vi "Live Image Test.vi"() -> ()   [LabVIEW 2017]
uses:
  <vilib>/vision/NI_Vision_Development_Module.lvlib
panel:
  in  "IP Address":string="192.168.0.90"
  out "HSL Image":T1(plugin-control)
  in  "Debug":bool
  out "Mono Image":T1(plugin-control)
  in  "Track":bool
  in  "Tracking":enum16{"None", "Color", "Circle", "Rect"}(ring)
  in  "Camera Op":T2(ring)=enum."JPG-CGI"
  in  "Acquire Params":T3={"fps"=10, "Compress"=30, "X Size"=320, "Y Size"=240, "Color?"=TRUE, "Rotation"=enum."0"}
  out "Waveform Chart":u32(graph)
  out "dT":u32
  in  "stop":bool
  out "Image":T1(plugin-control)
  out "Objects":i32
  # "Camera"
  # "Vision"
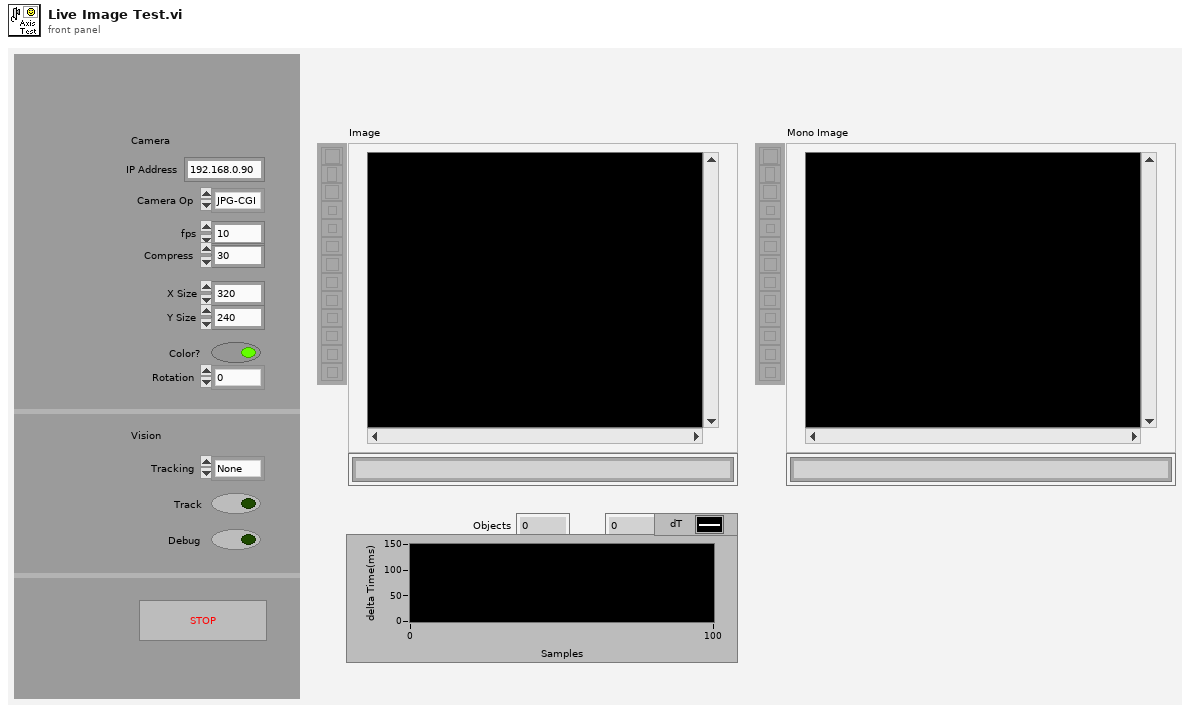
[diagram p1: front panel]
types:
  T1 = typedef "IMAQ Image.ctl" = refnum<image>
  T2 = enum16{"MJPG", "JPG", "JPG-CGI", "BMP", "BMP-CGI"}
  T3 = cluster{"fps":i32, "Compress":i32, "X Size":i32, "Y Size":i32, "Color?":bool, "Rotation":enum16{"0", "90", "180", "270"}}
  T4 = typedef "Image Type" = u32
  T5 = typedef "IMAQ ExtractCurvesCurve.ctl" = cluster{"Points":cluster{"X":dbl, "Y":dbl}[], "Closed?":bool, "Curve Length":dbl, "Min Edge Strength":dbl, "Max Edge Strength":dbl, "Average Edge Strength":dbl}
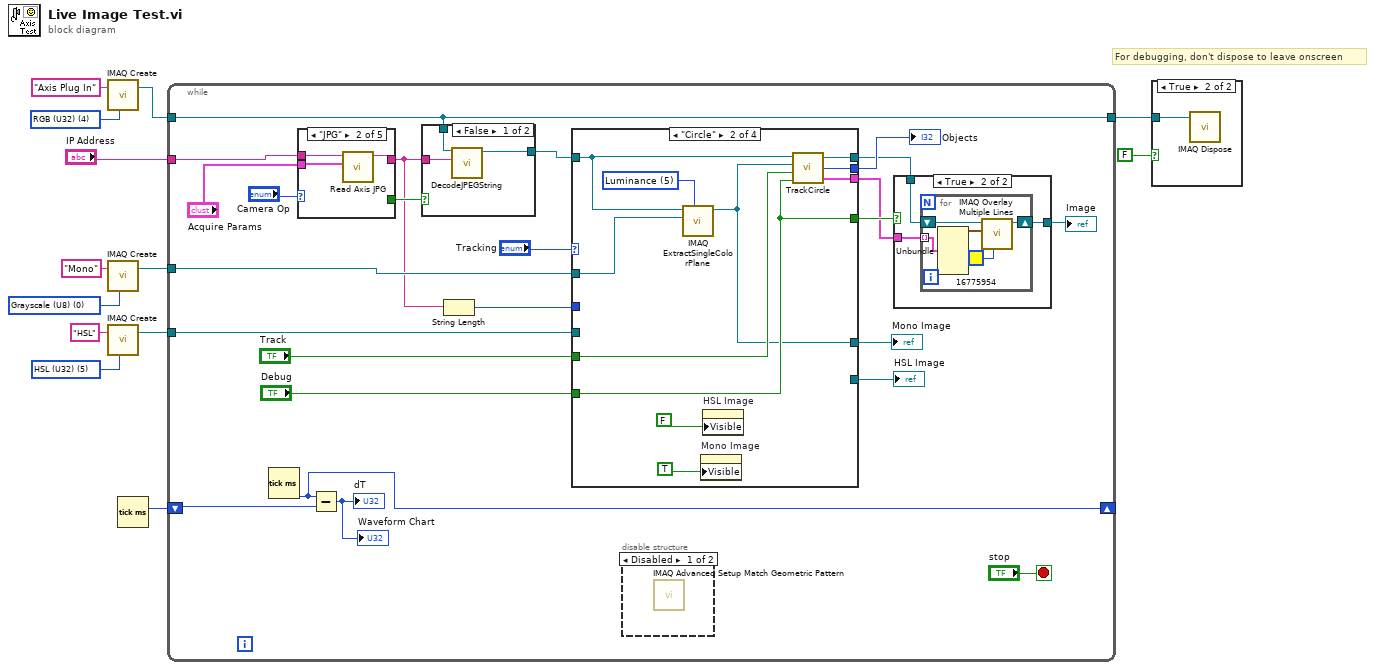
[diagram p0: block diagram]
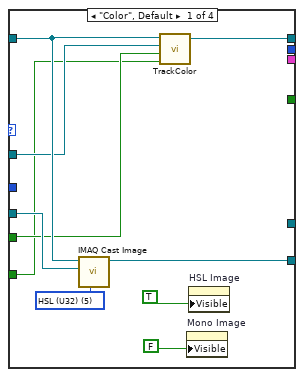
[diagram p5: hidden frame]
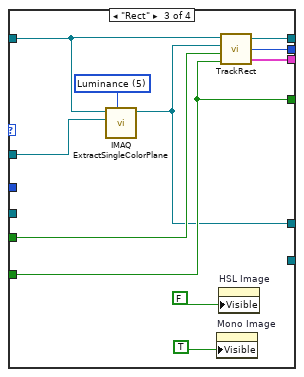
[diagram p6: hidden frame]
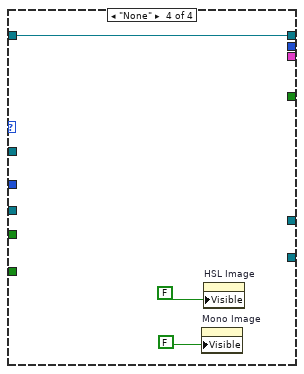
[diagram p7: hidden frame]
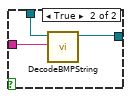
[diagram p8: hidden frame]
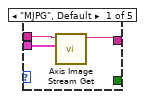
[diagram p9: hidden frame]
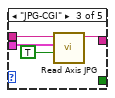
[diagram p10: hidden frame]
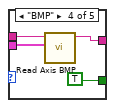
[diagram p11: hidden frame]
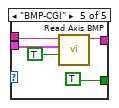
[diagram p12: hidden frame]
diagram:
  w2 = T4 5 items=["Grayscale (U8)", "Grayscale (I16)", "Grayscale (SGL)", "Complex (CSG)", "RGB (U32)", "HSL (U32)", "RGB (U64)"] ("Image Type")
  w6 = T4 0 items=["Grayscale (U8)", "Grayscale (I16)", "Grayscale (SGL)", "Complex (CSG)", "RGB (U32)", "HSL (U32)", "RGB (U64)"] ("Image Type")
  w7 = T4 4 items=["Grayscale (U8)", "Grayscale (I16)", "Grayscale (SGL)", "Complex (CSG)", "RGB (U32)", "HSL (U32)", "RGB (U64)"] ("Image Type")
  # "For debugging, don't dispose to leave onscreen"
  n1 = call "IMAQ Create"("Image Name"="Axis Plug In", "Image Type"=w7) -> ("New Image"=w12:T1)  [unwired: 3 in, 1 out]
  n2 = call "IMAQ Create"("Image Name"="Mono", "Image Type"=w6) -> ("New Image"=w4:T1)  [unwired: 3 in, 1 out]
  n3 = call "IMAQ Create"("Image Name"="HSL", "Image Type"=w2) -> ("New Image"=w1:T1)  [unwired: 3 in, 1 out]
  n4 = Tick Count (ms)() -> (millisecond timer value=w11:u32)
  n5 = while {
    tunnel: w12 -> [w33]
    shift-right: [w35] -> _
    shift-left: w11 -> [w36]
    tunnel: [w33] -> w10
    tunnel: "IP Address" -> [w30]
    tunnel: w4 -> [w27]
    tunnel: w1 -> [w14]
    stop <- "stop" stop-if-true
    n6 = Tick Count (ms)() -> (millisecond timer value=w35:u32)
    n7 = case shown="\"JPG\"" "Camera Op" {
      tunnel: w30 -> [w90 w93 w97 w101 w105]
      tunnel: [w89 w92 w96 w100 w106] -> w23
      tunnel: "Acquire Params" -> [w88 w91 w95 w99 w104]
      tunnel: [_ _ _ TRUE TRUE] -> w31
      frame "MJPG", Default {
        n8 = call <vilib>:"Axis Image Stream Get.vi"("Acquire Params"=w88, "IP Address"=w90) -> ("Raw Image Data"=w89:string)  [unwired: 9 in]
      }
      frame "JPG" {
        n9 = call <vilib>:"Read Axis JPG.vi"("Acquire Params"=w91, "address"=w93) -> ("Raw Image Data"=w92:string)  [unwired: 8 in, 1 out]
      }
      frame "JPG-CGI" {
        n10 = call <vilib>:"Read Axis JPG.vi"("CGI?"=TRUE, "Acquire Params"=w95, "address"=w97) -> ("Raw Image Data"=w96:string)  [unwired: 7 in, 1 out]
      }
      frame "BMP" {
        n11 = call <vilib>:"Read Axis BMP.vi"("Acquire Params"=w99, "address"=w101) -> ("Raw Image Data"=w100:string)  [unwired: 8 in, 1 out]
      }
      frame "BMP-CGI" {
        n12 = call <vilib>:"Read Axis BMP.vi"("CGI?"=TRUE, "Acquire Params"=w104, "address"=w105) -> ("Raw Image Data"=w106:string)  [unwired: 7 in, 1 out]
      }
    }
    n13 = Subtract(x=w35, y=w36) -> (x-y=→"dT" →"Waveform Chart":u32)
    n14 = case shown="False" w31 {
      tunnel: [w84 w86] -> w28
      tunnel: w33 -> [w83 w87]
      tunnel: w23 -> [w82 w85]
      frame False {
        n15 = call <vilib>:"DecodeJPEGString.vi"("Compressed Image"=w82, "Image In"=w83) -> ("Image Out"=w84:T1)  [unwired: 4 in, 1 out]
      }
      frame True {
        n16 = call <vilib>:"DecodeBMPString.vi"("Compressed Image"=w85, "Image In"=w87) -> ("Image Out"=w86:T1)  [unwired: 4 in, 1 out]
      }
    }
    n17 = String Length(string=w23) -> (length=w22:i32)
    n18 = case shown="\"Circle\"" "Tracking" {
      tunnel: w28 -> [w51 w66 w77 w81]
      tunnel: [w50 w67 w78 w81] -> w19
      tunnel: w27 -> [w49 w65 w76 _]
      tunnel: "Track" -> [w48 w64 w74 _]
      tunnel: [_ w62 w73 _] -> w25
      tunnel: w22 -> [_ _ _ _]
      tunnel: "Debug" -> [w47 w61 w71 _]
      tunnel: [_ w61 w71 _] -> w20
      tunnel: [_ w60 w72 _] -> w17
      tunnel: [_ w59 w70 _] -> w16
      tunnel: [w56 _ _ _] -> w15
      tunnel: w14 -> [w52 _ _ _]
      frame "Color", Default {
        w55 = T4 5 items=["Grayscale (U8)", "Grayscale (I16)", "Grayscale (SGL)", "Complex (CSG)", "RGB (U32)", "HSL (U32)", "RGB (U64)"] ("Image Type")
        n19 = call "IMAQ Cast Image"("Image Type"=w55, "Image Dst"=w52, "Image Src"=w51) -> ("Image Dst Out"=w56:T1)  [unwired: 7 in, 1 out]
        n20 = call <vilib>:"TrackColor.vi"("Debug"=w47, "Track"=w48, "Mono Image In 2"=w49, "Color Image In"=w51) -> ("ColorImage Out"=w50:T1)  [unwired: 1 in, 1 out]
        n21 = property on="Mono Image" class="ImageControl"("Visible"=FALSE) -> ()  [unwired: 2 in, 2 out]
        n22 = property on="HSL Image" class="ImageControl"("Visible"=TRUE) -> ()  [unwired: 2 in, 2 out]
      }
      frame "Circle" {
        w63 = 5 items=["Red", "Green", "Blue", "Hue", "Saturation", "Luminance", "Value", "Intensity"] ("Color Plane")
        n23 = call "IMAQ ExtractSingleColorPlane"("Color Plane"=w63, "Image Dst"=w65, "Image Src"=w66) -> ("Image Dst Out"=w59:T1)  [unwired: 7 in, 1 out]
        n24 = property on="Mono Image" class="ImageControl"("Visible"=TRUE) -> ()  [unwired: 2 in, 2 out]
        n25 = property on="HSL Image" class="ImageControl"("Visible"=FALSE) -> ()  [unwired: 2 in, 2 out]
        n26 = call <vilib>:"TrackCircle.vi"("Debug"=w61, "Track"=w64, "Mono Image In 2"=w59, "Color Image In"=w66) -> ("Curves"=w60:T5[], "Circles"=w62:i32, "ColorImage Out"=w67:T1)
      }
      frame "Rect" {
        w75 = 5 items=["Red", "Green", "Blue", "Hue", "Saturation", "Luminance", "Value", "Intensity"] ("Color Plane")
        n27 = call "IMAQ ExtractSingleColorPlane"("Color Plane"=w75, "Image Dst"=w76, "Image Src"=w77) -> ("Image Dst Out"=w70:T1)  [unwired: 7 in, 1 out]
        n28 = property on="Mono Image" class="ImageControl"("Visible"=TRUE) -> ()  [unwired: 2 in, 2 out]
        n29 = property on="HSL Image" class="ImageControl"("Visible"=FALSE) -> ()  [unwired: 2 in, 2 out]
        n30 = call <vilib>:"TrackRect.vi"("Debug"=w71, "Track"=w74, "Mono Image In 2"=w70, "Color Image In"=w77) -> ("Curves"=w72:T5[], "Rects"=w73:i32, "ColorImage Out"=w78:T1)
      }
      frame "None" {
        n31 = property on="Mono Image" class="ImageControl"("Visible"=FALSE) -> ()  [unwired: 2 in, 2 out]
        n32 = property on="HSL Image" class="ImageControl"("Visible"=FALSE) -> ()  [unwired: 2 in, 2 out]
      }
    }
    "Objects" <- w25
    "Mono Image" <- w16
    "HSL Image" <- w15
    n33 = disable-structure shown="Disabled" {
      frame Disabled {
        n34 = call "IMAQ Advanced Setup Match Geometric Pattern"() -> ()  [unwired: 9 in, 2 out]
      }
      frame Enabled {
      }
    }
    n35 = case shown="True" w20 {
      tunnel: w19 -> [w38 w41]
      tunnel: [w38 w40] -> w18
      tunnel: w17 -> [_ w39]
      frame False {
      }
      frame True {
        n36 = for {
          tunnel: w39 -> [w44] mode=indexing
          shift-right: [w45] -> w40
          shift-left: w41 -> [w46]
          n37 = Unbundle(w44) -> ("Points"=w43:cluster{"X":dbl, "Y":dbl}[])  [unwired: 5 out]
          n38 = call "IMAQ Overlay Multiple Lines"("Color"=u32 16775954, "Line End Points"=w43, "Image"=w46) -> ("Image Out"=w45:T1)  [unwired: 7 in, 1 out]
        }
      }
    }
    "Image" <- w18
  }
  n39 = case shown="True" FALSE {
    tunnel: w10 -> [_ w107]
    frame False {
    }
    frame True {
      n40 = call "IMAQ Dispose"("Image"=w107) -> ()  [unwired: 5 in, 1 out]
    }
  }
